vi "camera.vi"(5 "Media Source":string="rtsp://user:password@*.*.*.*/axis-media/media.amp?videocodec=h264", 11 "error in (no error)":errorcluster) -> (15 "error out":errorcluster)   [LabVIEW 2012]
uses:
  System.Windows.Forms
panel:
  in  "PictureBox":refnum<k24>(container)
  # "http://www.videolan.org/developers/vlc/doc/doxygen/html/modules.html"
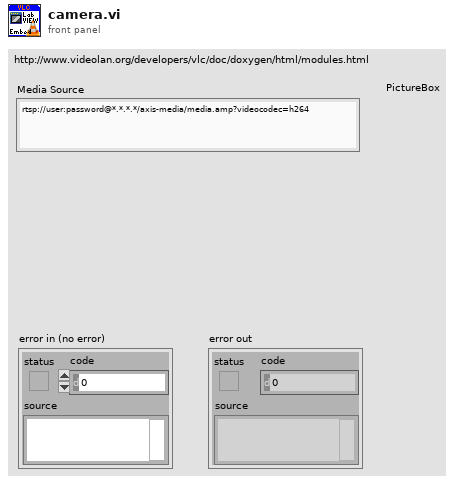
[diagram p1: front panel]
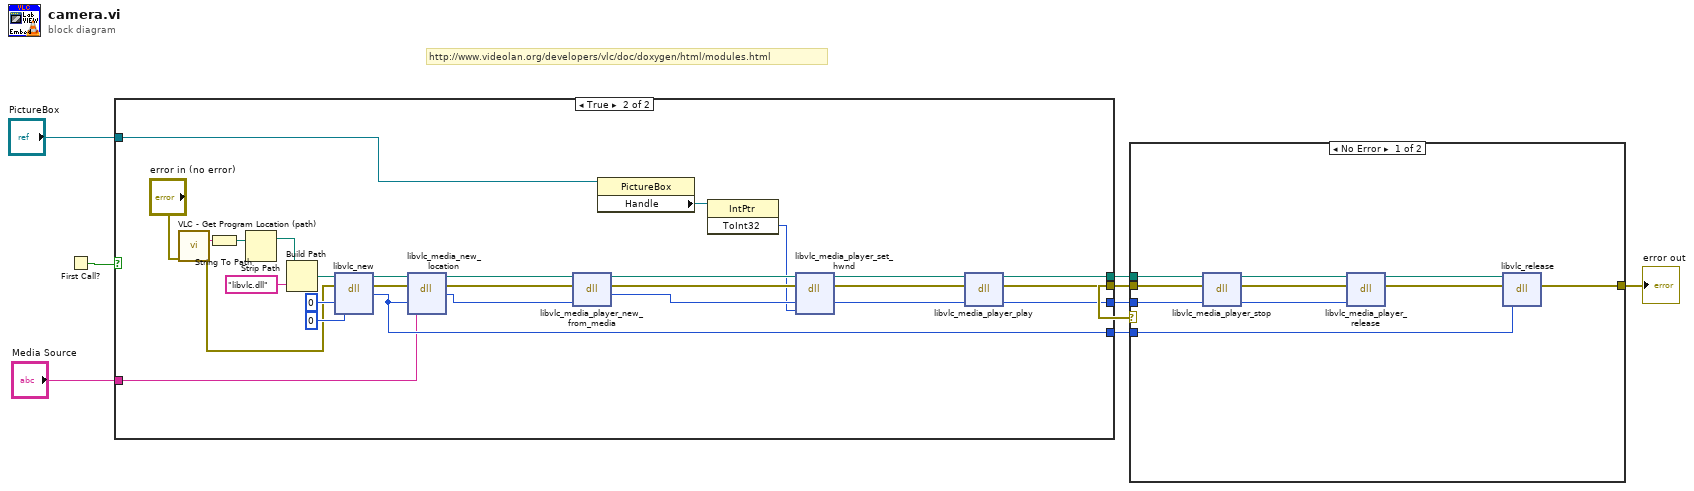
[diagram p0: block diagram]
diagram:
  # "http://www.videolan.org/developers/vlc/doc/doxygen/html/modules.html"
  n1 = First Call?() -> (First Call?: T/F=w1:bool)
  n2 = case shown="True" w1 {
    tunnel: [_ w36] -> w8
    tunnel: [_ w35] -> w7
    tunnel: [_ w24] -> w6
    tunnel: "Media Source" -> [_ w18]
    tunnel: [_ w15] -> w3
    tunnel: "PictureBox" -> [_ w13]
    frame False {
    }
    frame True {
      n3 = call "VLC - Get Program Location (path).vi"("error in (no error)"="error in (no error)") -> ("VLC path"=w23:string, "error out"=w16:errorcluster)  [unwired: 13 in]
      n4 = String To Path(string=w23) -> (path=w22:path)
      n5 = Strip Path(path=w22) -> (stripped path=w21:path)  [unwired: 1 out]
      n6 = Build Path(base path=w21, name or relative path="libvlc.dll") -> (appended path=w19:path)
      n7 = dll-call lib="C:/Program Files (x86)/VideoLAN/VLC/libvlc.dll" fn="libvlc_new"(path in=w19, error in=w16, "argc"=i16 0, "argv"=u8 0) -> (path out=w27:path, error out=w30:errorcluster, "return type"=w36:i32)  [unwired: 3 in]
      n8 = dll-call lib="C:/Program Files (x86)/VideoLAN/VLC/libvlc.dll" fn="libvlc_media_new_location"(path in=w27, error in=w30, "p_instance"=w36, "path"=w18) -> (path out=w14:path, error out=w10:errorcluster, "return type"=w9:i32)  [unwired: 3 in]
      n9 = dll-call lib="C:/Program Files (x86)/VideoLAN/VLC/libvlc.dll" fn="libvlc_media_player_new_from_media"(path in=w14, error in=w10, "p_md"=w9) -> (path out=w26:path, error out=w33:errorcluster, "return type"=w31:i32)  [unwired: 2 in]
      n10 = property class="PictureBox"(reference=w13) -> ("Handle"=w12:refnum<k24>)  [unwired: 1 in, 2 out]
      n11 = invoke class="IntPtr" method="ToInt32"(reference=w12) -> ("ToInt32"=w11:i32)  [unwired: 2 in, 2 out]
      n12 = dll-call lib="C:/Program Files (x86)/VideoLAN/VLC/libvlc.dll" fn="libvlc_media_player_set_hwnd"(path in=w26, error in=w33, "p_mi"=w31, "drawable"=w11) -> (path out=w25:path, error out=w34:errorcluster, "p_mi"=w32:i32)  [unwired: 3 in]
      n13 = dll-call lib="C:/Program Files (x86)/VideoLAN/VLC/libvlc.dll" fn="libvlc_media_player_play"(path in=w25, error in=w34, "p_mi"=w32) -> (path out=w24:path, error out=w15:errorcluster, "p_mi"=w35:i32)  [unwired: 2 in]
    }
  }
  n14 = case shown="No Error" w3 {
    tunnel: w8 -> [w46 _]
    tunnel: w7 -> [w45 _]
    tunnel: w3 -> [w44 w47]
    tunnel: w6 -> [w43 _]
    tunnel: [w42 w47] -> w4
    frame No Error {
      n15 = dll-call lib="C:/Program Files (x86)/VideoLAN/VLC/libvlc.dll" fn="libvlc_media_player_stop"(path in=w43, error in=w44, "p_mi"=w45) -> (path out=w38:path, error out=w41:errorcluster, "p_mi"=w40:i32)  [unwired: 2 in]
      n16 = dll-call lib="C:/Program Files (x86)/VideoLAN/VLC/libvlc.dll" fn="libvlc_media_player_release"(path in=w38, error in=w41, "p_mi"=w40) -> (path out=w37:path, error out=w39:errorcluster)  [unwired: 3 in]
      n17 = dll-call lib="C:/Program Files (x86)/VideoLAN/VLC/libvlc.dll" fn="libvlc_release"(path in=w37, error in=w39, "p_instnace"=w46) -> (error out=w42:errorcluster)  [unwired: 3 in, 1 out]
    }
    frame Error {
    }
  }
  "error out" <- w4
